vi "Configure Trigger (Pulse Width).vi"(0 "VISA resource name":refnum<visa-resource-name>, 1 "Trigger Condition (0: Less Than)":u16(ring) items=["Less Than", "More Than", "Equal", "Not Equal"], 2 "Pulse Width (4.0ns)":dbl=4e-09, 5 "Trigger Source (0: Channel 1)":u16(ring) items=["Channel 1"=0, "Channel 2"=1, "Channel 3"=2, "Channel 4"=3, "AC Line"=11, "Aux"=12, "Digital Channel 0"=14, "Digital Channel 1"=15, "Digital Channel 2"=16, "Digital Channel 3"=17, "Digital Channel 4"=18, "Digital Channel 5"=19, "Digital Channel 6"=20, "Digital Channel 7"=21, "Digital Channel 8"=22, "Digital Channel 9"=23, "Digital Channel 10"=24, "Digital Channel 11"=25, "Digital Channel 12"=26, "Digital Channel 13"=27, "Digital Channel 14"=28, "Digital Channel 15"=29], 7 "Trigger Threshold (0.0V)":dbl, 9 "Trigger Polarity (0: Positive)":u16(ring) items=["Positive", "Negative"], 11 "error in (no error)":errorcluster) -> (4 "VISA resource name out":refnum<visa-resource-name>, 15 "error out":errorcluster)   [LabVIEW 2013, in "Tektronix DPO MSO 2000 4000 Series.lvlib"]
doc: "Configures pulse width trigger settings for an oscilloscope. A pulse width trigger occurs when the trigger signal has a pulse with a width that meets the value you specify in <B>Trigger Condition</B>. The trigger does not occur until the edge of a pulse that corresponds to the pulse width polarity crosses the threshold you specify in <B>Trigger Level</B>."
uses:
  Tektronix DPO MSO 2000 4000 Series.lvlib
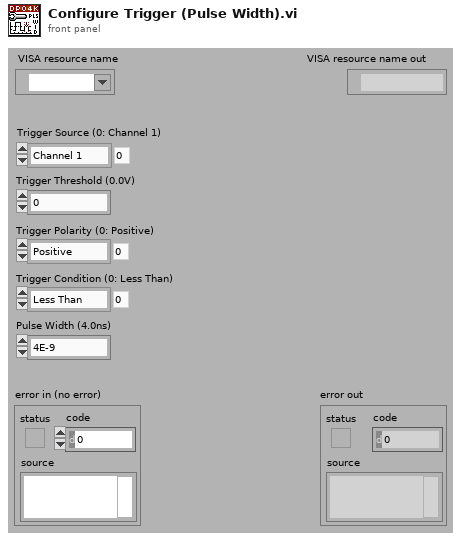
[diagram p1: front panel]
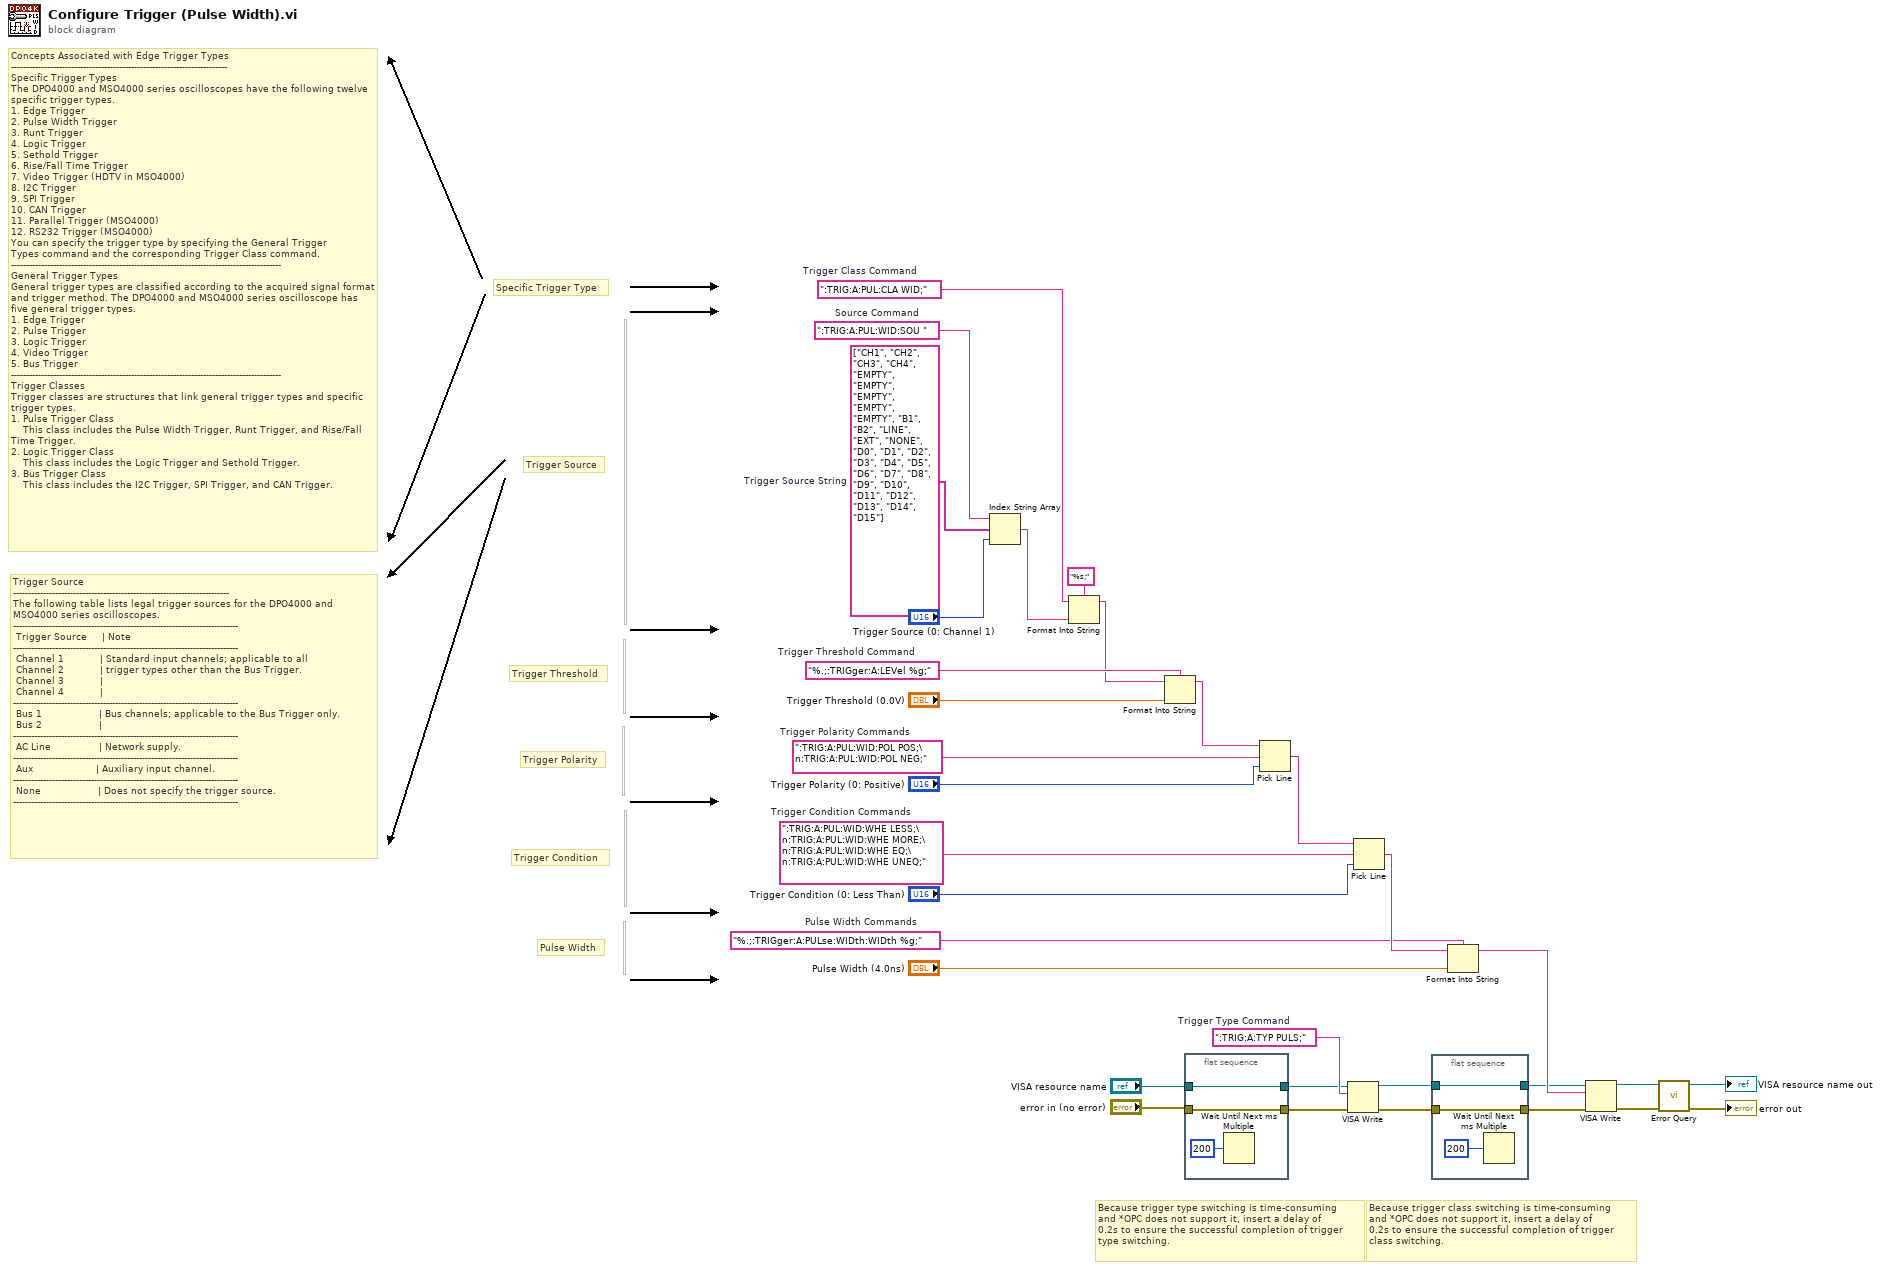
[diagram p0: block diagram]
diagram:
  w14 = string[] ["CH1", "CH2", "CH3", "CH4", "EMPTY", "EMPTY", "EMPTY", "EMPTY", "EMPTY", "B1", "B2", "LINE", "EXT", "NONE", "D0", "D1", "D2", "D3", "D4", "D5", "D6", "D7", "D8", "D9", "D10", "D11", "D12", "D13", "D14", "D15"]  # Trigger Source String
  w25 = "%.;:TRIGger:A:PULse:WIDth:WIDth %g;"  # Pulse Width Commands
  w19 = ":TRIG:A:PUL:WID:WHE LESS;\n:TRIG:A:PUL:WID:WHE MORE;\n:TRIG:A:PUL:WID:WHE EQ;\n:TRIG:A:PUL:WID:WHE UNEQ;"  # Trigger Condition Commands
  w17 = ":TRIG:A:PUL:WID:POL POS;\n:TRIG:A:PUL:WID:POL NEG;"  # Trigger Polarity Commands
  w15 = "%.;:TRIGger:A:LEVel %g;"  # Trigger Threshold Command
  w32 = ":TRIG:A:PUL:WID:SOU "  # Source Command
  w13 = ":TRIG:A:PUL:CLA WID;"  # Trigger Class Command
  w22 = ":TRIG:A:TYP PULS;"  # Trigger Type Command
  # "Trigger Source\n------------------------------------------------------------------------\nThe following table lists legal trigger sources for the DPO4000 and MSO4000 series oscilloscopes.\n---------------------------------------------------------------------------\n Trigger Source     | Note                                                           \n---------------------------------------------------------------------------\n Channel 1            | Standard input channels; applicable to all      \n Channel 2            | trigger types other than the Bus Trigger.         \n Channel 3            |     \n Channel 4            |\n---------------------------------------------------------------------------\n Bus 1                   | Bus channels; applicable to the Bus Trigger only.\n Bus 2                   | \n---------------------------------------------------------------------------\n AC Line                | Network supply.\n---------------------------------------------------------------------------\n Aux                     | Auxiliary input channel.\n---------------------------------------------------------------------------\n None                   | Does not specify the trigger source.\n---------------------------------------------------------------------------"
  # "Concepts Associated with Edge Trigger Types\n------------------------------------------------------------------------\nSpecific Trigger Types\nThe DPO4000 and MSO4000 series oscilloscopes have the following twelve specific trigger types.\n1. Edge Trigger\n2. Pulse Width Trigger\n3. Runt Trigger\n4. Logic Trigger\n5. Sethold Trigger\n6. Rise/Fall Time Trigger\n7. Video Trigger (HDTV in MSO4000)\n8. I2C Trigger\n9. SPI Trigger\n10. CAN Trigger\n11. Parallel Trigger (MSO4000)\n12. RS232 Trigger (MSO4000)\nYou can specify the trigger type by specifying the General Trigger \nTypes command and the corresponding Trigger Class command.\n------------------------------------------------------------------------------------------\nGeneral Trigger Types \nGeneral trigger types are classified according to the acquired signal format and trigger method. The DPO4000 and MSO4000 series oscilloscope has five general trigger types.\n1. Edge Trigger\n2. Pulse Trigger\n3. Logic Trigger\n4. Video Trigger\n5. Bus Trigger\n------------------------------------------------------------------------------------------\nTrigger Classes\nTrigger classes are structures that link general trigger types and specific trigger types.\n1. Pulse Trigger Class\n    This class includes the Pulse Width Trigger, Runt Trigger, and Rise/Fall Time Trigger.\n2. Logic Trigger Class\n    This class includes the Logic Trigger and Sethold Trigger.\n3. Bus Trigger Class\n    This class includes the I2C Trigger, SPI Trigger, and CAN Trigger."
  # "Because trigger class switching is time-consuming\nand *OPC does not support it, insert a delay of\n0.2s to ensure the successful completion of trigger\nclass switching."
  # "Because trigger type switching is time-consuming\nand *OPC does not support it, insert a delay of\n0.2s to ensure the successful completion of trigger\ntype switching."
  # "Trigger Polarity"
  # "Pulse Width"
  # "Trigger Condition"
  # "Trigger Threshold"
  # "Trigger Source"
  # "Specific Trigger Type"
  n1 = Index String Array(1:"Trigger Source (0: Channel 1)", 2:w14, 3:w32) -> (0:w30:string)
  n2 = Format Into String(format string="%s;", initial string=w13, w30) -> (resulting string=w12:string)  [unwired: 1 in, 1 out]
  n3 = Format Into String(format string=w15, initial string=w12, "Trigger Threshold (0.0V)") -> (resulting string=w11:string)  [unwired: 1 in, 1 out]
  n4 = flat-sequence {
    tunnel: "VISA resource name" -> [w34]
    tunnel: [w34] -> w21
    tunnel: "error in (no error)" -> [w33]
    tunnel: [w33] -> w20
    frame #0 {
      n5 = Wait Until Next ms Multiple(millisecond multiple=u32 200) -> ()  [unwired: 1 out]
    }
  }
  n6 = Pick Line(string ("")=w11, multi-line string=w17, line index="Trigger Polarity (0: Positive)") -> (output string=w10:string)
  n7 = VISA Write(VISA resource name=w21, write buffer=w22, error in (no error)=w20) -> (VISA resource name out=w24:refnum<visa-resource-name>, error out=w23:errorcluster)  [unwired: 1 out]
  n8 = Pick Line(string ("")=w10, multi-line string=w19, line index="Trigger Condition (0: Less Than)") -> (output string=w26:string)
  n9 = flat-sequence {
    tunnel: w24 -> [w36]
    tunnel: [w37] -> w7
    tunnel: w23 -> [w37]
    tunnel: [w36] -> w8
    frame #0 {
      n10 = Wait Until Next ms Multiple(millisecond multiple=u32 200) -> ()  [unwired: 1 out]
    }
  }
  n11 = Format Into String(format string=w25, initial string=w26, "Pulse Width (4.0ns)") -> (resulting string=w9:string)  [unwired: 1 in, 1 out]
  n12 = VISA Write(VISA resource name=w8, write buffer=w9, error in (no error)=w7) -> (VISA resource name out=w6:refnum<visa-resource-name>, error out=w5:errorcluster)  [unwired: 1 out]
  n13 = call "Error Query.vi"("error in (no error)"=w5, "VISA resource name"=w6) -> ("error out"=→"error out":errorcluster, "VISA resource name out"=→"VISA resource name out":refnum<visa-resource-name>)  [unwired: 6 in, 2 out]
